vi "Keithley Control Panel 2.vi"(8 "error in":T2) -> (0 "error out":T2, 2 "Reading Numerical Result":dbl)   [LabVIEW 2017]
uses:
  Global/GPIB Numbers.vi
panel:
  out "String":string
  in  "Rate (ms)":i32=100
  in  "integ. value":dbl=0.01667 format="%^.2e"
  in  "integration time (0:auto)":u16(ring) items=["automatic", "automatic once", "set to minimum", "set to maximum", "set aperature value", "set NPLC value"]
  in  "digital filter (off:0)":u16(ring) items=["off", "auto filter", "auto filter once", "moving filter", "repeating filter"]
  in  "dig. filter count":dbl=10.0 min=1.0 max=100.0 step=1.0 format="%^.2e"
  in  "range (auto:0)":u16(ring) items=["autorange", "autorange once", "set min range", "set max range", "set range value"]
  in  "reference (off:0)":u16(ring) items=["off", "set reference value"]
  in  "noise tolerance (%)":dbl=1.0 min=0.0 max=100.0 step=1.0 format="%^.2e"
  in  "resolution (4.5 digits:3)":u16(ring)=3 items=["auto resolution", "auto resolution once", "3.5 digits", "4.5 digits", "5.5 digits", "6.5 digits", "7.5 digits", "8.5 digits"]
  in  "advanced filter (off:0)":u16(ring) items=["off", "enabled"]
  in  "coupling":bool=TRUE
  in  "Tab Control":T1(tab) caption="Select the Keithly mode to us"
  in  "range value (volts)":dbl=750.0 min=0.2 max=750.0 format="%^.2e"
  in  "reference value (volts)":dbl min=-775.0 max=775.0 format="%^.2e"
  in  "AC voltage (volts:0)":u16(ring) items=["volts", "DB", "DBM"]
  in  "dB reference (volts)":dbl=1.0 min=0.001 max=750.0 format="%.3f"
  in  "detector (rms:0)":u16(ring) items=["RMS", "average", "low frequency RMS", "AC peak voltage", "DC negative peak spike", "DC positive peak spike"]
  in  "peak window (secs)":dbl=0.1 min=0.1 max=9.9 format="%.2f"
  in  "dBm ref impedance (75:1)":u16(ring)=1 items=["50 ohms", "75 ohms", "93 ohms", "132 ohms", "300 ohms", "600 ohms"]
  in  "range value (volts)":dbl=1000.0 min=0.2 max=1000.0 format="%^.2e"
  in  "reference value (volts)":dbl min=-1100.0 max=1100.0 format="%^.2e"
  in  "range value (ohms)":dbl=1000000000.0 min=20.0 max=1000000000.0 format="%^.2e"
  in  "reference value (ohms)":dbl min=-1000000000.0 max=1000000000.0 format="%^.2e"
  in  "offset compensation":bool
  in  "range value (ohms)":dbl=200000.0 min=20.0 max=200000.0 format="%^.2e"
  in  "reference value (ohms)":dbl min=-200000.0 max=200000.0 format="%^.2e"
  in  "offset compensation":bool
  in  "range value (amps)":dbl=2.0 min=0.0002 max=2.0 format="%^.2e"
  in  "reference value (amps)":dbl min=-2.1 max=2.1 format="%^.2e"
  in  "detector (rms:0)":u16(ring) items=["RMS", "average"]
  in  "range value (amps)":dbl=2.0 min=0.0002 max=2.0 format="%^.2e"
  in  "method":bool=TRUE
  in  "reference value (amps)":dbl min=-2.1 max=2.1 format="%^.2e"
  in  "threshold voltage level":dbl min=-600.0 max=600.0 step=1.0 format="%^.2e"
  in  "threshold voltage range (10V:1)":u16(ring)=1 items=["1 V", "10 V", "100 V", "1000 V", "TTL"]
  in  "threshold current level":dbl min=-0.6 max=0.6 format="%^.2e"
  in  "reference value (Hz)":dbl min=0.0 max=15000000.0 format="%^.2e"
  in  "threshold current range (1mA:0)":u16(ring) items=["1 mA", "10 mA", "100 mA", "1 A"]
  in  "resolution (5 digits:1)":u16(ring)=1 items=["4 digits", "5 digits"]
  in  "source":bool
  in  "Set Values":bool
  in  "stop":bool
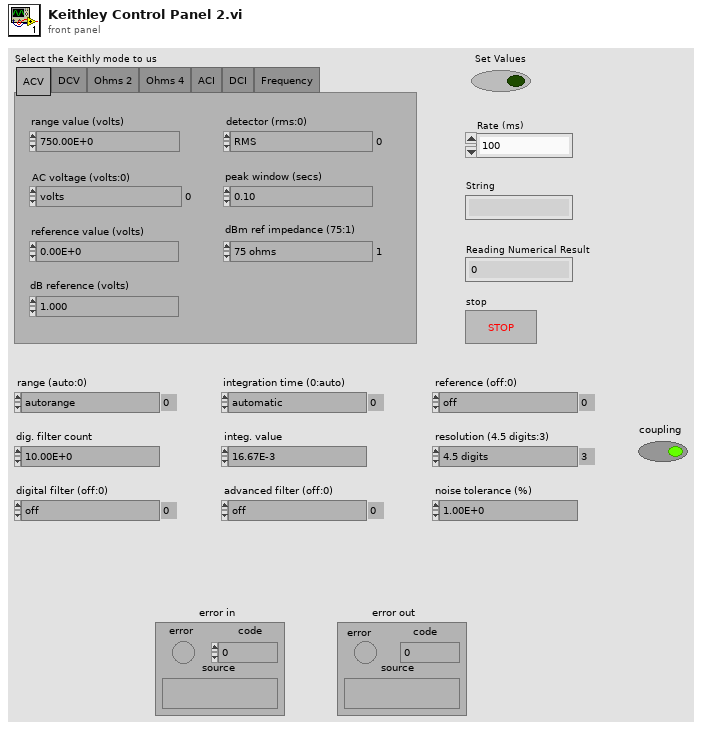
[diagram p1: front panel]
types:
  T1 = enum32{"ACV", "DCV", "Ohms 2", "Ohms 4", "ACI", "DCI", "Frequency"}
  T2 = cluster{"error":bool, "code":i32, "source":string}
  T3 = typedef "GPIB Type Def.ctl" = cluster{"Name":string, "bus":dbl, "GPIB":dbl, "GPIB as string":string, "byte":i32, "VISA Resource Name":refnum<visa-resource-name>}
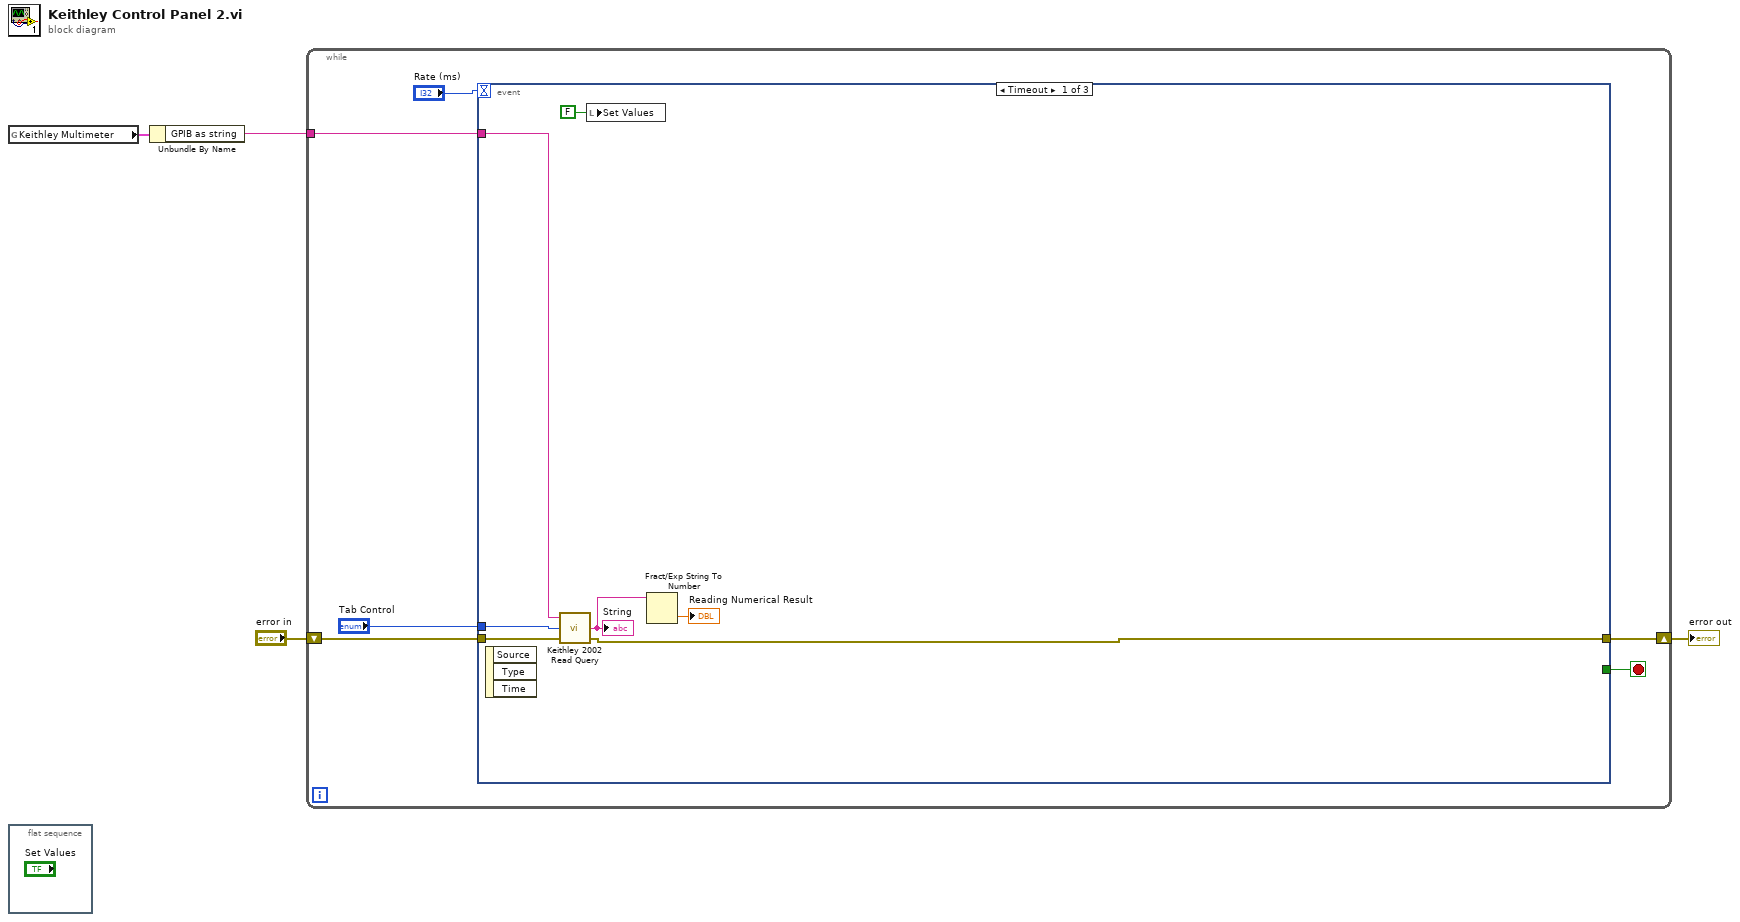
[diagram p0: block diagram]
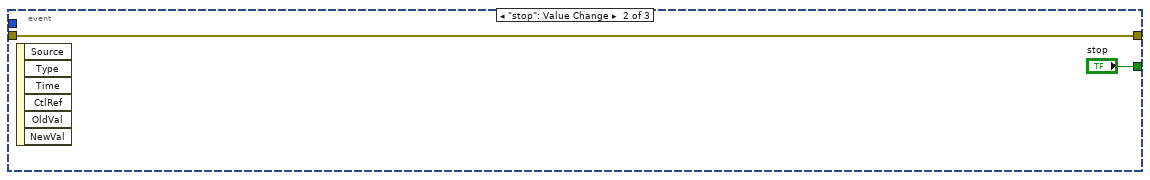
[diagram p2: hidden frame]
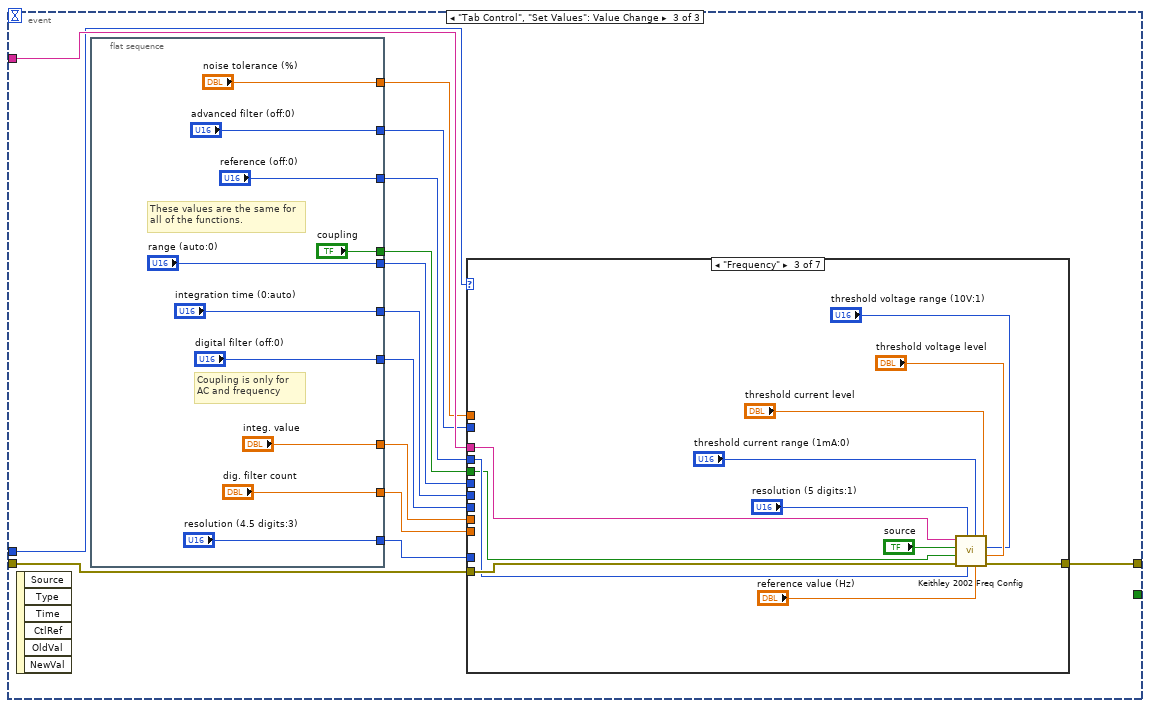
[diagram p3: hidden frame]
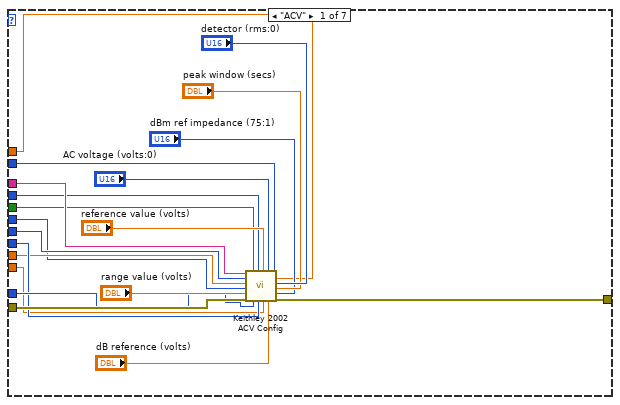
[diagram p4: hidden frame]
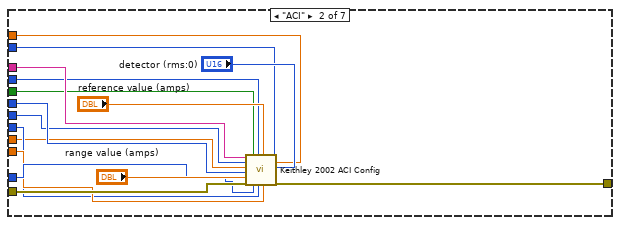
[diagram p5: hidden frame]
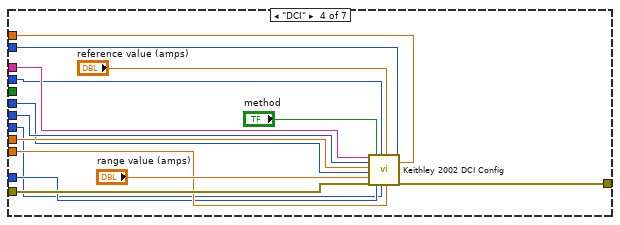
[diagram p6: hidden frame]
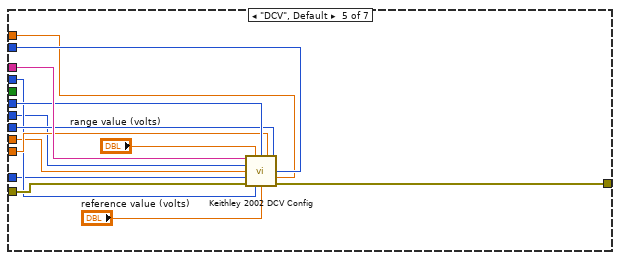
[diagram p7: hidden frame]
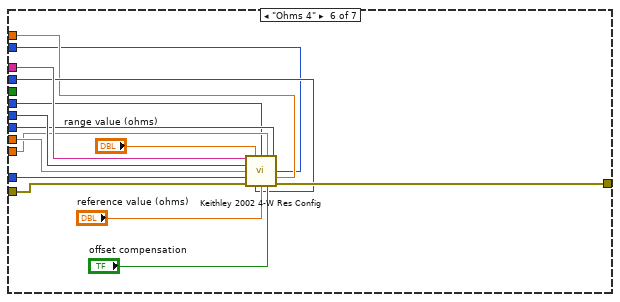
[diagram p8: hidden frame]
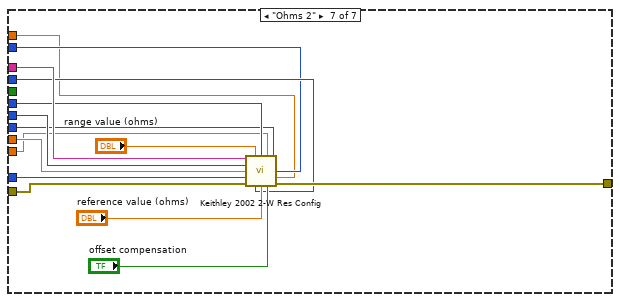
[diagram p9: hidden frame]
diagram:
  n1 = global read "GPIB Numbers.vi" "Keithley Multimeter"() -> (w4:T3)
  n2 = flat-sequence {
    frame #0 {
    }
  }
  n3 = Unbundle By Name(w4) -> ("GPIB as string"=w2:string)
  n4 = while {
    shift-right: [w6] -> w3
    shift-left: "error in" -> [w8]
    tunnel: w2 -> [w9]
    stop <- w10 stop-if-true
    n5 = event shown="[0] Timeout" {
      selector: _ -> [_ _ _]
      dyn-events: _ -> [_ _ _]
      timeout: "Rate (ms)" -> [_ _ _]
      tunnel: w8 -> [w13 w18 w33]
      tunnel: [w12 w18 w30] -> w6
      tunnel: [_ "stop" _] -> w10
      tunnel: w9 -> [w15 _ w32]
      tunnel: "Tab Control" -> [w11 _ w31]
      event Timeout {
        n6 = event-data() -> ()  [unwired: 1 in, 3 out]
        n7 = call "Keithley 2002 Read Query.vi"("error in"=w13, "function (Vdc:1)"=w11, "GPIB Address"=w15) -> ("error out"=w12:T2, "Reading Result"=w14:string)  [unwired: 1 in]
        "String" <- w14
        n8 = local write "Set Values"(FALSE ("Set Values")) -> ()
        n9 = Fract/Exp String To Number(string=w14) -> (number=→"Reading Numerical Result":dbl)  [unwired: 3 in, 1 out]
      }
      event "stop": Value Change {
        n10 = event-data() -> ()  [unwired: 1 in, 6 out]
      }
      event "Tab Control", "Set Values": Value Change {
        n11 = event-data() -> ()  [unwired: 1 in, 6 out]
        n12 = flat-sequence {
          tunnel: ["reference (off:0)"] -> w27
          tunnel: ["integration time (0:auto)"] -> w21
          tunnel: ["range (auto:0)"] -> w23
          tunnel: ["dig. filter count"] -> w26
          tunnel: ["digital filter (off:0)"] -> w25
          tunnel: ["noise tolerance (%)"] -> w29
          tunnel: ["advanced filter (off:0)"] -> w28
          tunnel: ["integ. value"] -> w22
          tunnel: ["resolution (4.5 digits:3)"] -> w24
          tunnel: ["coupling"] -> w20
          frame #0 {
            # "Coupling is only for \nAC and frequency"
            # "These values are the same for\nall of the functions."
          }
        }
        n13 = case shown="\"Frequency\"" w31 {
          tunnel: w33 -> [w63 w79 w90 w106 w120 w134 w150]
          tunnel: w32 -> [w61 w77 w91 w104 w118 w135 w149]
          tunnel: [w62 w78 w89 w105 w119 w133 w148] -> w30
          tunnel: w24 -> [w53 w70 _ w93 w107 w127 w144]
          tunnel: w25 -> [w52 w68 _ w92 w113 w123 w138]
          tunnel: w29 -> [w46 w73 _ w100 w111 w125 w136]
          tunnel: w28 -> [w51 w72 _ w97 w112 w124 w137]
          tunnel: w27 -> [w50 w71 w81 w98 w110 w126 w143]
          tunnel: w21 -> [w49 w65 _ w96 w109 w129 w141]
          tunnel: w22 -> [w48 w66 _ w95 w108 w128 w142]
          tunnel: w23 -> [w47 w67 _ w94 w115 w121 w140]
          tunnel: w26 -> [w45 w69 _ w99 w114 w122 w139]
          tunnel: w20 -> [w44 w64 w80 _ _ _ _]
          frame "ACV" {
            n14 = call "Keithley 2002 ACV Config.vi"("GPIB address"=w61, "integration time (0:auto)"=w49, "integ. value"=w48, "range (auto:0)"=w47, "range value (volts)"="range value (volts)", "error in"=w63, "coupling"=w44, "resolution (4.5 digits:3)"=w53, "reference (off:0)"=w50, "digital filter (off:0)"=w52, "reference value (volts)"="reference value (volts)", "dig. filter count"=w45, "AC voltage (volts:0)"="AC voltage (volts:0)", "dB reference (volts)"="dB reference (volts)", "advanced filter (off:0)"=w51, "noise tolerance (%)"=w46, "detector (rms:0)"="detector (rms:0)", "peak window (secs)"="peak window (secs)", "dBm ref impedance (75:1)"="dBm ref impedance (75:1)") -> ("error out"=w62:T2)
          }
          frame "ACI" {
            n15 = call "Keithley 2002 ACI Config.vi"("GPIB address"=w77, "integration time (0:auto)"=w65, "integ. value"=w66, "range (auto:0)"=w67, "range value (amps)"="range value (amps)", "error in"=w79, "coupling"=w64, "resolution (4.5 digits:3)"=w70, "reference (off:0)"=w71, "digital filter (off:0)"=w68, "reference value (amps)"="reference value (amps)", "dig. filter count"=w69, "advanced filter (off:0)"=w72, "noise tolerance (%)"=w73, "detector (rms:0)"="detector (rms:0)") -> ("error out"=w78:T2)  [unwired: 4 in]
          }
          frame "Frequency" {
            n16 = call "Keithley 2002 Freq Config.vi"("threshold voltage level"="threshold voltage level", "threshold voltage range (10V:1)"="threshold voltage range (10V:1)", "threshold current level"="threshold current level", "reference value (Hz)"="reference value (Hz)", "threshold current range (1mA:0)"="threshold current range (1mA:0)", "reference (off:0)"=w81, "resolution (5 digits:1)"="resolution (5 digits:1)", "error in"=w90, "coupling"=w80, "source"="source", "GPIB address"=w91) -> ("error out"=w89:T2)
          }
          frame "DCI" {
            n17 = call "Keithley 2002 DCI Config.vi"("GPIB address"=w104, "integration time (0:auto)"=w96, "integ. value"=w95, "range (auto:0)"=w94, "range value (amps)"="range value (amps)", "error in"=w106, "method"="method", "resolution (4.5 digits:3)"=w93, "reference (off:0)"=w98, "digital filter (off:0)"=w92, "reference value (amps)"="reference value (amps)", "dig. filter count"=w99, "advanced filter (off:0)"=w97, "noise tolerance (%)"=w100) -> ("error out"=w105:T2)  [unwired: 5 in]
          }
          frame "DCV", Default {
            n18 = call "Keithley 2002 DCV Config.vi"("GPIB address"=w118, "range value (volts)"="range value (volts)", "range (auto:0)"=w115, "dig. filter count"=w114, "digital filter (off:0)"=w113, "integration time (0:auto)"=w109, "integ. value"=w108, "advanced filter (off:0)"=w112, "resolution (4.5 digits:3)"=w107, "noise tolerance (%)"=w111, "error in"=w120, "reference (off:0)"=w110, "reference value (volts)"="reference value (volts)") -> ("error out"=w119:T2)  [unwired: 2 in]
          }
          frame "Ohms 4" {
            n19 = call "Keithley 2002 4-W Res Config.vi"("GPIB address"=w135, "range value (ohms)"="range value (ohms)", "range (auto:0)"=w121, "dig. filter count"=w122, "digital filter (off:0)"=w123, "integration time (0:auto)"=w129, "integ. value"=w128, "advanced filter (off:0)"=w124, "resolution (4.5 digits:3)"=w127, "noise tolerance (%)"=w125, "error in"=w134, "reference (off:0)"=w126, "reference value (ohms)"="reference value (ohms)", "offset compensation"="offset compensation") -> ("error out"=w133:T2)  [unwired: 1 in]
          }
          frame "Ohms 2" {
            n20 = call "Keithley 2002 2-W Res Config.vi"("GPIB address"=w149, "range value (ohms)"="range value (ohms)", "range (auto:0)"=w140, "dig. filter count"=w139, "digital filter (off:0)"=w138, "integration time (0:auto)"=w141, "integ. value"=w142, "advanced filter (off:0)"=w137, "resolution (4.5 digits:3)"=w144, "noise tolerance (%)"=w136, "error in"=w150, "reference (off:0)"=w143, "reference value (ohms)"="reference value (ohms)", "offset compensation"="offset compensation") -> ("error out"=w148:T2)  [unwired: 1 in]
          }
        }
      }
    }
  }
  "error out" <- w3
